vi "index from range.vi"(8 "left":dbl, 10 "right":dbl, 11 "omega":dbl[](array[numeric])) -> (0 "left index":dbl, 1 "length":dbl, 2 "right index":dbl)   [LabVIEW 2018]
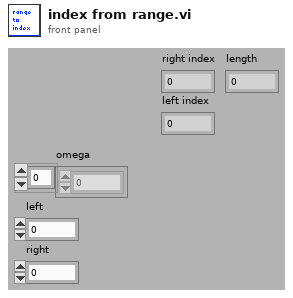
[diagram p1: front panel]
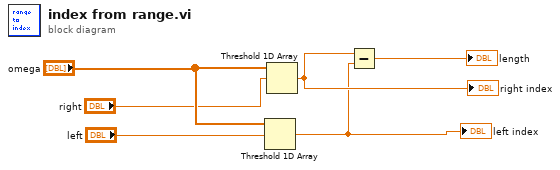
[diagram p0: block diagram]
diagram:
  n1 = Threshold 1D Array(2:"left", 3:"omega") -> (0:w1:dbl)  [unwired: 1 in]
  "left index" <- w1
  n2 = Threshold 1D Array(2:"right", 3:"omega") -> (0:w5:dbl)  [unwired: 1 in]
  "right index" <- w5
  n3 = Subtract(x=w5, y=w1) -> (x-y=→"length":dbl)
